vi "Generic Camera Get New Image.vi"(0 "Camera Notifier Name":string) -> (8 "Image Out":u16[][](array[numeric]))   [LabVIEW 2025]
uses:
  <vilib>/vision/Image Controls.llb/IMAQ Image.ctl
  Camera Controls/Generic Camera Actions.ctl
  Microscope Modules/4Pi Objective Image Alignment/4Pi OIA - Controls/4Pi OIA - ROI Selection.ctl
  Camera Controls/Camera IMAQ Key Info.ctl
  Display Module/Display Module Custom Controls/ROI Descriptor.ctl
panel:
  in  "Image Ref":T1
  in  "Frame Accums.":u16
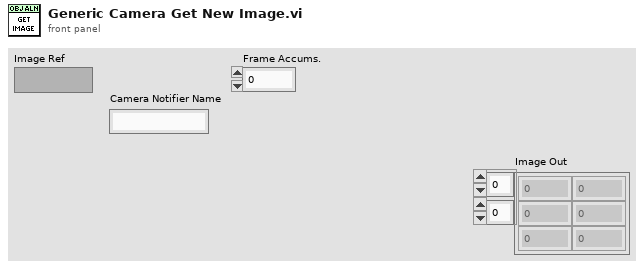
[diagram p1: front panel]
types:
  T1 = typedef "IMAQ Image.ctl" = refnum<image>
  T2 = typedef "4Pi OIA - ROI Selection.ctl" = enum32{"Full Image", "ROI"}
  T3 = typedef "Generic Camera Actions.ctl" = enum16{"Status", "Live Preview", "Capture", "Abort", "Set Exposure Time (s)", "Get Exposure Time (s)", "Record Settings", "Binning", "Set ROI", "Get ROI", "Defect Correction On?", "Cooler On?", "Fan On?", "Quit"}
  T4 = typedef "ROI Descriptor.ctl" = cluster{"Global Rectangle":i32[], "Contours":cluster{"Contour Type":u32, "ROI Type":u32, "Points":i32[]}[]}
  T5 = typedef "Camera IMAQ Key Info.ctl" = cluster{"Frame":u32, "Sensor Height":i32, "Sensor Width":i32, "ROI Height":i32, "ROI Width":i32, "ROI Enable?":bool, "Bit per Pixel":u8}
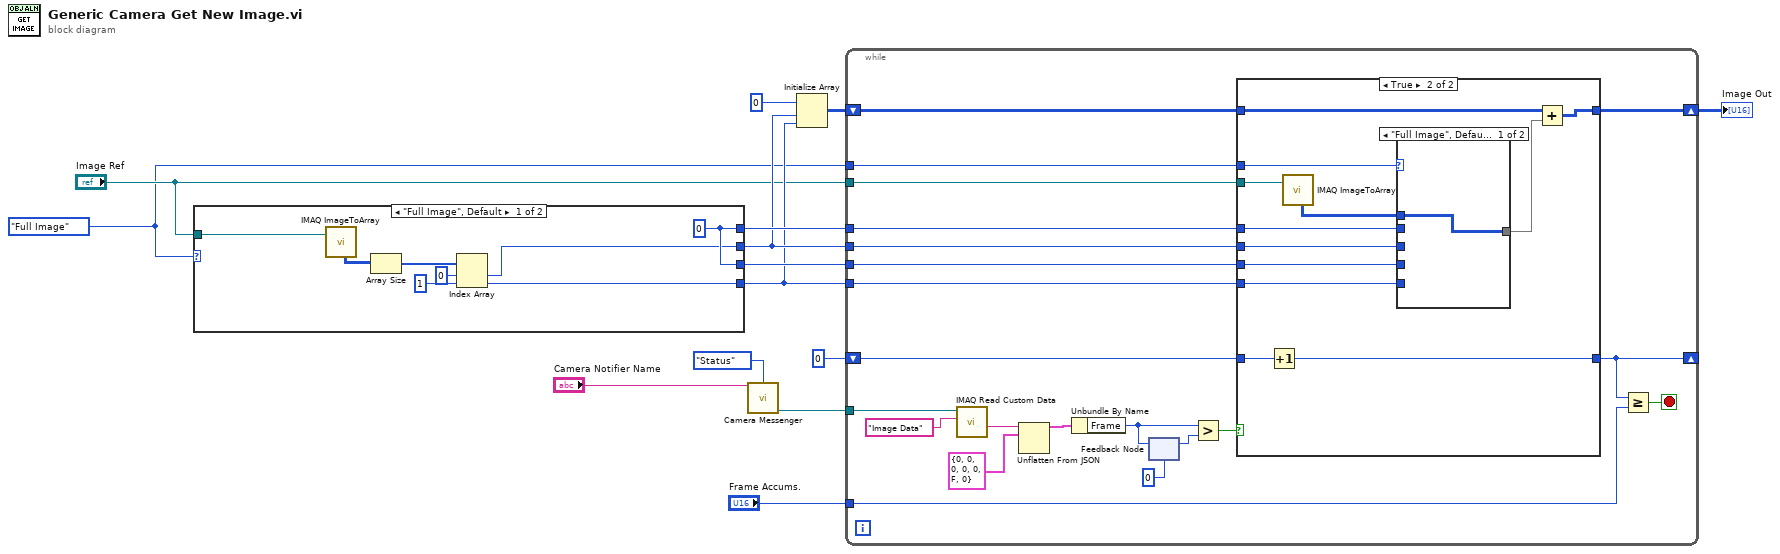
[diagram p0: block diagram]
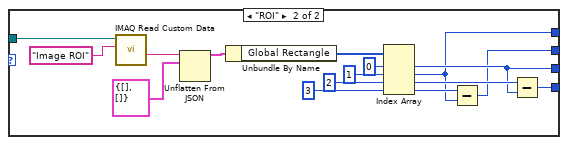
[diagram p2: hidden frame]
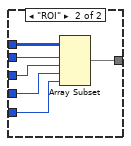
[diagram p4: hidden frame]
diagram:
  w1 = 4Pi_OIA_-_ROI_Selection."Full Image" ("ROI Selection")
  n1 = case shown="\"Full Image\", Default" w1 {
    tunnel: "Image Ref" -> [w21 w29]
    tunnel: [w22 w26] -> w8
    tunnel: [w15 w25] -> w6
    tunnel: [w22 w24] -> w9
    tunnel: [w16 w23] -> w7
    frame "Full Image", Default {
      w22 = 0
      n2 = call "IMAQ ImageToArray"("Image"=w21) -> ("Image Pixels (U16)"=w20:u16[][])  [unwired: 3 in, 4 out]
      n3 = Array Size(array=w20) -> (size(s)=w19:i32[])
      n4 = Index Array(array=w19, index #1=0 ("index"), index #2=1 ("index")) -> (element #1=w16:i32, element #2=w15:i32)
    }
    frame "ROI" {
      n5 = call "IMAQ Read Custom Data"("Key"="Image ROI", "Image"=w29) -> ("Custom Data Out"=w37:string)  [unwired: 7 in, 2 out]
      n6 = Unflatten From JSON(JSON string=w37, type and defaults=T4 {"Global Rectangle"=[], "Contours"=[]} ("Image ROI Descriptor")) -> (value=w35:T4)  [unwired: 5 in, 1 out]
      n7 = Unbundle By Name(w35) -> ("Global Rectangle"=w34:i32[])
      n8 = Index Array(array=w34, index #1=0 ("index"), index #2=1 ("index"), index #3=2 ("index"), index #4=3 ("index")) -> (element #1=w26:i32, element #2=w24:i32, element #3=w27:i32, element #4=w28:i32)
      n9 = Subtract(x=w28, y=w24) -> (x-y=w23:i32)
      n10 = Subtract(x=w27, y=w26) -> (x-y=w25:i32)
    }
  }
  n11 = call "Camera Messenger.vi"("Notifier Name"="Camera Notifier Name", "General Camera Actions"=Generic_Camera_Actions."Status") -> ("Image Ref"=w13:T1)  [unwired: 8 in, 5 out]
  n12 = Initialize Array(u16 0, w7, w6) -> (w11:u16[][])
  n13 = while {
    tunnel: w13 -> [w55]
    shift-right: [w49] -> _
    shift-left: u16 0 -> [w50]
    tunnel: w1 -> [w47]
    tunnel: "Image Ref" -> [w46]
    shift-right: [w40] -> w5
    shift-left: w11 -> [w41]
    tunnel: w9 -> [w45]
    tunnel: w7 -> [w44]
    tunnel: w8 -> [w43]
    tunnel: w6 -> [w42]
    tunnel: "Frame Accums." -> [w39]
    stop <- w48 stop-if-true
    n14 = call "IMAQ Read Custom Data"("Key"="Image Data", "Image"=w55) -> ("Custom Data Out"=w57:string)  [unwired: 7 in, 2 out]
    n15 = Unflatten From JSON(JSON string=w57, type and defaults=T5 {"Frame"=0, "Sensor Height"=0, "Sensor Width"=0, "ROI Height"=0, "ROI Width"=0, "ROI Enable?"=FALSE, "Bit per Pixel"=0} ("Camera IMAQ Key Info")) -> (value=w59:T5)  [unwired: 5 in, 1 out]
    n16 = Unbundle By Name(w59) -> ("Frame"=w52:u32)
    n17 = feedback #1(u32 0 ("Frame")) -> (w54:u32)
    n18 = feedback-in #1(w52) -> ()
    n19 = Greater?(x=w52, y=w54) -> (0:w51:bool)
    n20 = case shown="True" w51 {
      tunnel: w50 -> [w61 w73]
      tunnel: [w61 w72] -> w49
      tunnel: w47 -> [_ w71]
      tunnel: w46 -> [_ w70]
      tunnel: w45 -> [_ w68]
      tunnel: w44 -> [_ w67]
      tunnel: w43 -> [_ w66]
      tunnel: w42 -> [_ w65]
      tunnel: w41 -> [w60 w64]
      tunnel: [w60 w62] -> w40
      frame False {
      }
      frame True {
        n21 = Increment(x=w73) -> (x+1=w72:u16)
        n22 = call "IMAQ ImageToArray"("Image"=w70) -> ("Image Pixels (U16)"=w69:u16[][])  [unwired: 3 in, 4 out]
        n23 = case shown="\"Full Image\", Default" w71 {
          tunnel: w69 -> [w74 w80]
          tunnel: w68 -> [_ w79]
          tunnel: w67 -> [_ w78]
          tunnel: w66 -> [_ w77]
          tunnel: w65 -> [_ w76]
          tunnel: [w74 w75] -> w63
          frame "Full Image", Default {
          }
          frame "ROI" {
            n24 = Array Subset(array=w80, index (row)=w79, length (row)=w78, index (col)=w77, length (col)=w76) -> (w75:u16[][])
          }
        }
        n25 = Add(x=w64, y=w63) -> (x+y=w62:u16[][])
      }
    }
    n26 = Greater Or Equal?(x=w49, y=w39) -> (x >= y?=w48:bool)
  }
  "Image Out" <- w5
